vi "FadeOldFRFs.vi"(11 "WaveformGraph in":refnum<vi>) -> ()   [LabVIEW 2022 SP3]
uses:
  Mic/Mic_Global.vi
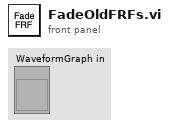
[diagram p1: front panel]
types:
  T1 = cluster{"Alerts":bool, "Log X Axis":bool, "dB scale":bool, "Averaging":bool, "Fade":dbl, "Centroids?":bool}
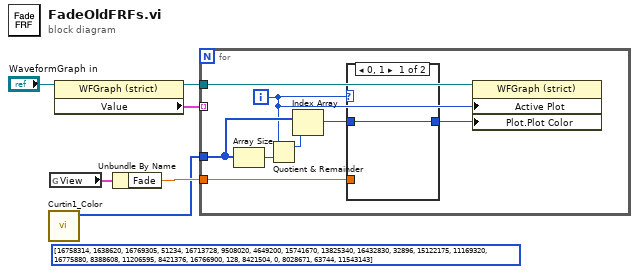
[diagram p0: block diagram]
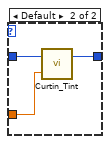
[diagram p2: hidden frame]
diagram:
  (unwired) u32[] [16758314, 1638620, 16769305, 51234, 16713728, 9508020, 4649200, 15741670, 13825340, 16432830, 32896, 15122175, 11169320, 16775880, 8388608, 11206595, 8421376, 16766900, 128, 8421504, 0, 8028671, 63744, 11543143] ("Colors")
  n1 = call "Curtin1_Color.vi"() -> ("Color palette"=w1:u32[])  [unwired: 10 in, 1 out]
  n2 = global read "Mic_Global.vi" "View"() -> (w3:T1)
  n3 = property class="WFGraph (strict)"(reference="WaveformGraph in") -> (reference out=w5:refnum<vi>, "Value"=w4:cluster{dbl, "df":dbl, dbl[]}[])  [unwired: 1 in, 1 out]
  n4 = Unbundle By Name(w3) -> ("Fade"=w2:dbl)
  n5 = for {
    tunnel: w5 -> [w10]
    tunnel: w1 -> [w12]
    tunnel: w4 -> [_] mode=indexing
    tunnel: w2 -> [w9]
    i -> [w7]
    n6 = Array Size(array=w12) -> (size(s)=w11:i32)
    n7 = Quotient & Remainder(x=w7, y=w11) -> (x-y*floor(x/y)=w13:i32)  [unwired: 1 out]
    n8 = Index Array(array=w12, index=w13) -> (element=w14:u32)
    n9 = case shown="0, 1" w7 {
      tunnel: w14 -> [w15 w18]
      tunnel: w9 -> [_ w17]
      tunnel: [w15 w16] -> w8
      frame 0, 1 {
      }
      frame Default {
        n10 = call "Curtin_Tint.vi"("Tint Factor"=w17, "Plot.Plot Color"=w18) -> ("Plot.Plot Color 2"=w16:u32)  [unwired: 1 in]
      }
    }
    n11 = property on="Property Node" class="WFGraph (strict)"(reference=w10, "Active Plot"=w7, "Plot.Plot Color"=w8) -> ()  [unwired: 1 in, 2 out]
  }
